vi "PH_DeformableMirror.SetChannelsZero.vi"(0 "i ref in":refnum<vi>, 5 "error in":errorcluster) -> (14 "i ref out":refnum<vi>, 19 "error out":errorcluster)   [LabVIEW 2014, in "PH_DeformableMirror.lvlib"]
uses:
  PH_DeformableMirror.lvlib
  instr.lib/dmdriver/DMirrorBase/DMirrorBase.lvclass
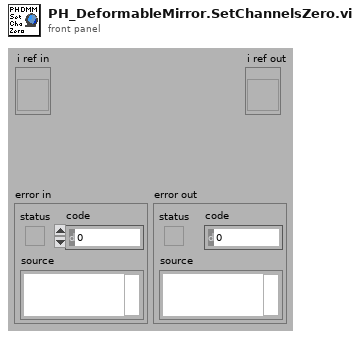
[diagram p1: front panel]
types:
  T1 = typedef "PH_DeformableMirror.lvlib/PH_DeformableMirror.i attribute.ctl" = cluster{"DMirror.lvlib:DMirrorBase.lvclass":refnum<class "DMirrorBase.lvclass">, "Device error":errorcluster, "GUI Refs":cluster{"Delete":refnum<vi>, "Device Error":refnum<vi>, "HV on":refnum<vi>, "Channel":refnum<vi>, "Voltage":refnum<vi>, "Channel Voltages":refnum<vi>}}
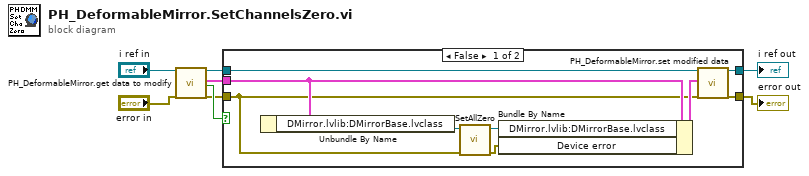
[diagram p0: block diagram]
diagram:
  n1 = call "PH_DeformableMirror.get data to modify.vi"("i ref in"="i ref in", "error in (no error)"="error in") -> ("i ref out"=w7:refnum<vi>, "i attribute"=w5:T1, "timed out"=w8:bool, "error out"=w6:errorcluster)  [unwired: 14 in]
  n2 = case shown="False" w8 {
    tunnel: [w17 w19] -> w4
    tunnel: w7 -> [w16 w19]
    tunnel: [w15 w18] -> w1
    tunnel: w6 -> [w9 w18]
    tunnel: w5 -> [w14 _]
    frame False {
      n3 = Unbundle By Name(w14) -> ("DMirror.lvlib:DMirrorBase.lvclass"=w13:refnum<class "DMirrorBase.lvclass">)
      n4 = call-dynamic "SetAllZero.vi"("error in (no error)"=w9, "DMirrorBase in"=w13) -> ("error out"=w10:errorcluster, "DMirrorBase out"=w11:refnum<class "DMirrorBase.lvclass">)  [unwired: 8 in]
      n5 = Bundle By Name(cluster=w14, "DMirror.lvlib:DMirrorBase.lvclass"=w11, "Device error"=w10) -> (w12:T1)
      n6 = call "PH_DeformableMirror.set modified data.vi"("i ref in"=w16, "i attribute"=w12, "error in (no error)"=w9) -> ("i ref out"=w17:refnum<vi>, "error out"=w15:errorcluster)  [unwired: 15 in]
    }
    frame True {
    }
  }
  "error out" <- w1
  "i ref out" <- w4
